vi "message_with_timestamp_CCP.vi"(8 "time_in":timestamp format="%<%Y-%m-%d %H:%M:%S>T", 11 "message_in":string="Message") -> (3 "message_out":string)   [LabVIEW 2019]
panel:
  out "time":timestamp format="%<%Y-%m-%d %H:%M:%S>T"
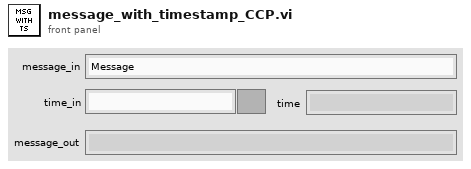
[diagram p1: front panel]
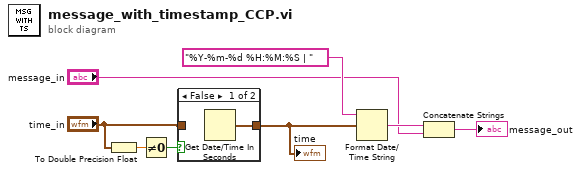
[diagram p0: block diagram]
diagram:
  n1 = To Double Precision Float(number="time_in") -> (double precision float=w8:dbl)
  n2 = Not Equal To 0?(x=w8) -> (x != 0?=w7:bool)
  n3 = case shown="False" w7 {
    tunnel: [w9 w10] -> w5
    tunnel: "time_in" -> [_ w10]
    frame False {
      n4 = Get Date/Time In Seconds() -> (seconds since 1Jan1904=w9:timestamp)
    }
    frame True {
    }
  }
  "time" <- w5
  n5 = Format Date/Time String(time format string (%c)="%Y-%m-%d %H:%M:%S | ", seconds (now)=w5) -> (date/time string=w3:string)  [unwired: 1 in]
  n6 = Concatenate Strings(w3, "message_in") -> (→"message_out":string)
